vi "File Create Wilt.vi"(0 "base path":path=path "c:/data", 2 "File Record Type":enum16{"History", "Sample", "Big Sample", ""}(ring)=enum."Big Sample", 5 "All Dryer Array In":T1[](array[typedef]) {"Night Cycle Count" format="%04d"; "Dryer Details"."Stop Dryer" items=["NO", "YES"]; "Dryer Details"."24 Hour Water Injection" items=["NO", "YES"]; "Dryer Details"."Run w/o Newfi" items=["NO", "YES"]; "Day Cycle Count" format="%04d"}, 7 "Single Dryer In":T1 {"Night Cycle Count" format="%04d"; "Dryer Details"."Stop Dryer" items=["NO", "YES"]; "Dryer Details"."24 Hour Water Injection" items=["NO", "YES"]; "Dryer Details"."Run w/o Newfi" items=["NO", "YES"]; "Day Cycle Count" format="%04d"}) -> (4 "appended path":path)   [LabVIEW 2012]
uses:
  Dryer.ctl
  Dryer Details.ctl
  Globals Wilt.vi
  <vilib>/Utility/file.llb/Write To Spreadsheet File (string).vi
panel:
  out "error out":errorcluster
  out "Array to Write":string[][](array[string])
  # "D"
  # "N"
  # "D"
  # "N"
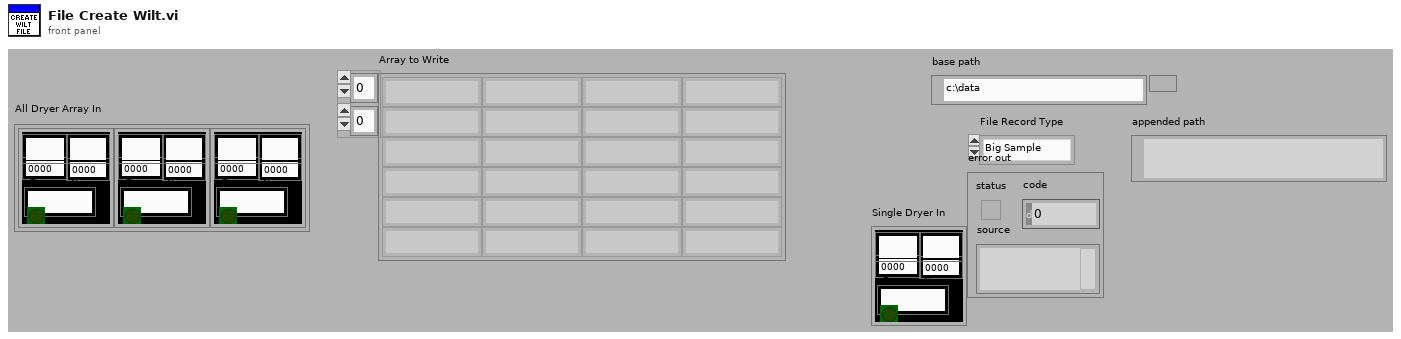
[diagram p1: front panel]
types:
  T1 = typedef "Dryer.ctl" = cluster{"Lab ID":string, "Day Cycle Count":i32, "Station Label":string, "Dryer Details":T2, "Sample Record ":string[], "Hist Record ":string[][], "Status Color":u32, "Boolean":bool, "Com Port":u8, "Bad Com Count":i32, "Current Run Start Time":dbl, "Night Cycle Count":i32, "Station Index":i32, "Cycle Index":string, "Audit Alert":bool}
  T2 = typedef "Dryer Details.ctl" = cluster{"Station":string, "Cycle Count Day":string, "Status":string, "Debug ASCII":string, "Notes":string, "Lab ID":string, "Total Time On":string, "TR Number":string, "Cycle Count Night":string, "Time On Day":string, "Time On Night":string, "Run w/o Newfi":i32, "24 Hour Water Injection":i32, "Stop Dryer":i32}
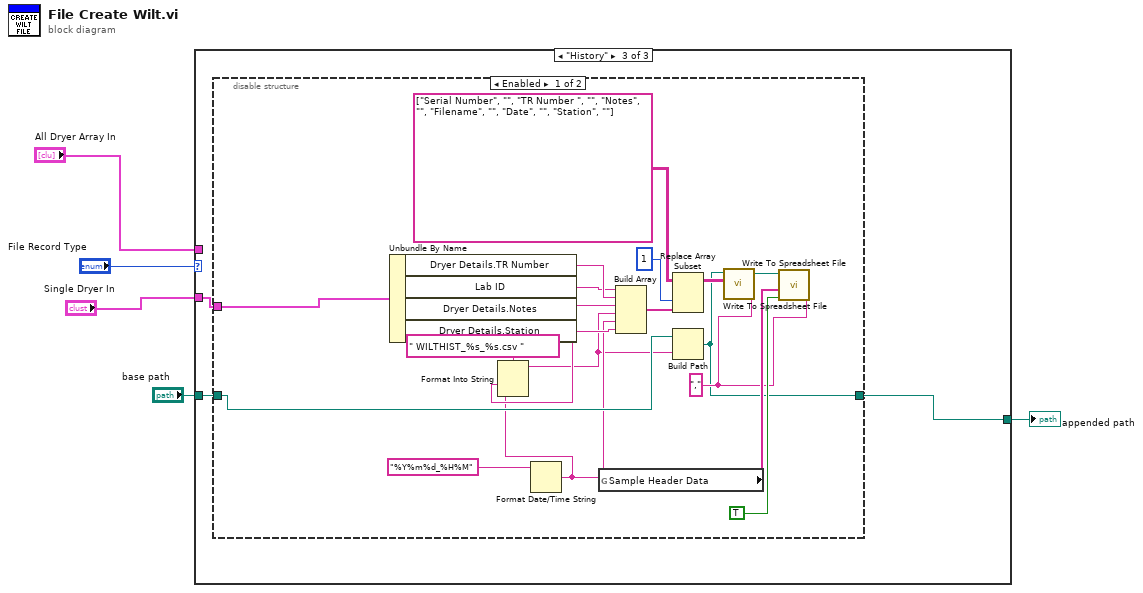
[diagram p0: block diagram]
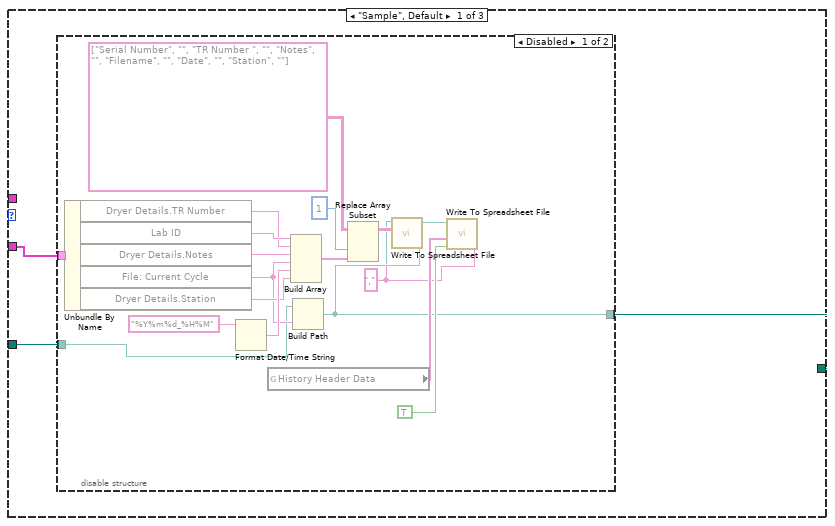
[diagram p2: hidden frame]
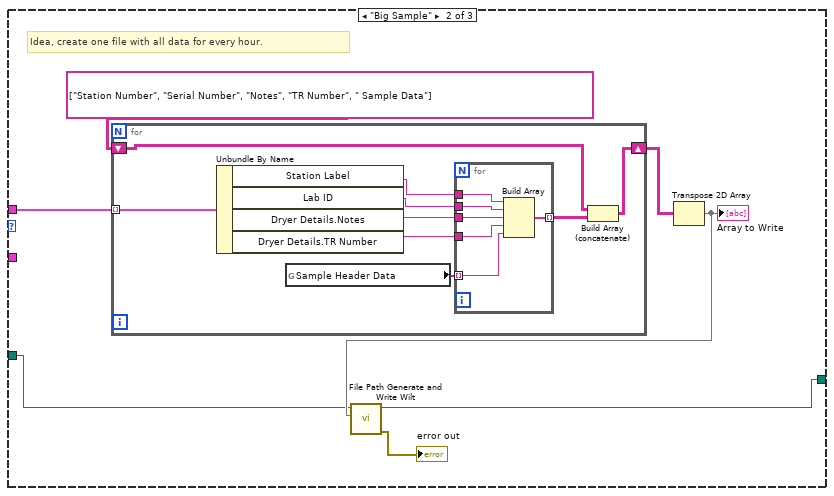
[diagram p4: hidden frame]
diagram:
  n1 = case shown="\"History\"" "File Record Type" {
    tunnel: "Single Dryer In" -> [w8 _ w51]
    tunnel: "base path" -> [w7 w28 w50]
    tunnel: [w6 w30 w49] -> w2
    tunnel: "All Dryer Array In" -> [_ w31 _]
    frame "Sample", Default {
      n2 = disable-structure shown="Disabled" {
        disable-tunnel: w8 -> [w15 _]
        disable-tunnel: w7 -> [w10 _]
        disable-tunnel: [w9 _] -> w6
        frame Disabled {
          w13 = "," ("delimiter (\\t)")
          n3 = Unbundle By Name(w15) -> ("Dryer Details.TR Number"=w23:string, "Lab ID"=w24:string, "Dryer Details.Notes"=w26:string, "File: Current Cycle"=w12:string, "Dryer Details.Station"=w14:string)
          n4 = Format Date/Time String(time format string (%c)="%Y%m%d_%H%M") -> (date/time string=w20:string)  [unwired: 2 out]
          n5 = global read "Globals Wilt.vi" "History Header Data"() -> (w16:string[])
          n6 = Build Array(w24, w23, w26, w12, w20, w14) -> (w22:string[])
          n7 = Build Path(base path=w10, name or relative path=w12) -> (appended path=w9:path)
          n8 = Replace Array Subset(array=string[][] [["Serial Number", ""], ["TR Number ", ""], ["Notes", ""], ["Filename", ""], ["Date", ""], ["Station", ""]], new element=w22, index (col)=1 ("disabled index (col)")) -> (w11:string[][])  [unwired: 1 in]
          n9 = call-poly <vilib>:"Write To Spreadsheet File.vi"("delimiter (\\t)"=w13, "2D data"=w11, "file path (dialog if empty)"=w9) -> ("new file path (Not A Path if cancelled)"=w17:path)  [unwired: 5 in]
          n10 = call-poly <vilib>:"Write To Spreadsheet File.vi"("delimiter (\\t)"=w13, "append to file? (new file:F)"=TRUE, "1D data"=w16, "file path (dialog if empty)"=w17) -> ()  [unwired: 4 in, 1 out]
        }
        frame Enabled {
        }
      }
    }
    frame "Big Sample" {
      # "Idea, create one file with all data for every hour."
      n11 = for {
        tunnel: w31 -> [w42] mode=indexing
        shift-right: [w38] -> w33
        shift-left: string[][] [["Station Number", "Serial Number", "Notes", "TR Number", " Sample Data"]] -> [w37]
        n12 = Unbundle By Name(w42) -> ("Station Label"=w34:string, "Lab ID"=w41:string, "Dryer Details.Notes"=w36:string, "Dryer Details.TR Number"=w35:string)
        n13 = global read "Globals Wilt.vi" "Sample Header Data"() -> (w40:string[])
        n14 = for {
          tunnel: w34 -> [w48]
          tunnel: w41 -> [w47]
          tunnel: [w46] -> w39 mode=indexing
          tunnel: w40 -> [w45] mode=indexing
          tunnel: w36 -> [w44]
          tunnel: w35 -> [w43]
          n15 = Build Array(w48, w47, w44, w43, w45) -> (w46:string[])
        }
        n16 = Build Array (concatenate)(w37, w39) -> (w38:string[][])
      }
      n17 = Transpose 2D Array(2D array=w33) -> (transposed array=w29:string[][])
      "Array to Write" <- w29
      n18 = call "File Path Generate and Write Wilt.vi"("Data Array"=w29, "base path"=w28) -> ("error out"=→"error out":errorcluster, "new file path (Not A Path if cancelled)"=w30:path)  [unwired: 8 in]
    }
    frame "History" {
      n19 = disable-structure shown="Enabled" {
        disable-tunnel: w51 -> [w61 _]
        disable-tunnel: w50 -> [w57 _]
        disable-tunnel: [w56 _] -> w49
        frame Enabled {
          w59 = "," ("delimiter (\\t)")
          n20 = Unbundle By Name(w61) -> ("Dryer Details.TR Number"=w68:string, "Lab ID"=w54:string, "Dryer Details.Notes"=w70:string, "Dryer Details.Station"=w60:string)
          n21 = Format Date/Time String(time format string (%c)="%Y%m%d_%H%M") -> (date/time string=w53:string)  [unwired: 2 out]
          n22 = Format Into String(format string=" WILTHIST_%s_%s.csv ", w54, w53) -> (resulting string=w52:string)  [unwired: 2 in, 1 out]
          n23 = global read "Globals Wilt.vi" "Sample Header Data"() -> (w62:string[])
          n24 = Build Array(w54, w68, w70, w52, w53, w60) -> (w67:string[])
          n25 = Replace Array Subset(array=string[][] [["Serial Number", ""], ["TR Number ", ""], ["Notes", ""], ["Filename", ""], ["Date", ""], ["Station", ""]], new element=w67, index (col)=1 ("disabled index (col)")) -> (w58:string[][])  [unwired: 1 in]
          n26 = Build Path(base path=w57, name or relative path=w52) -> (appended path=w56:path)
          n27 = call-poly <vilib>:"Write To Spreadsheet File.vi"("delimiter (\\t)"=w59, "2D data"=w58, "file path (dialog if empty)"=w56) -> ("new file path (Not A Path if cancelled)"=w63:path)  [unwired: 5 in]
          n28 = call-poly <vilib>:"Write To Spreadsheet File.vi"("delimiter (\\t)"=w59, "append to file? (new file:F)"=TRUE, "1D data"=w62, "file path (dialog if empty)"=w63) -> ()  [unwired: 4 in, 1 out]
        }
        frame Disabled {
        }
      }
    }
  }
  "appended path" <- w2
